vi "disable error reporting.vi"(8 "error in":errorcluster, 10 "module ID":string, 11 "Standard Engine Configuration in":refnum<class "Standard Engine Configuration.lvclass">) -> (0 "error out":errorcluster, 3 "Standard Engine Configuration out":refnum<class "Standard Engine Configuration.lvclass">)   [LabVIEW 2013, in "Standard Engine Configuration.lvclass"]
doc: "Undos the actions taken by the 'enable error reporting.vi'."
uses:
  Standard Engine Configuration.lvclass
  <vilib>/NI/Configuration Framework/serializable configuration/NISE_CEF_serializable configuration.lvclass/NISE_CEF_serializable configuration.ctl
  Standard Engine Configuration.lvclass/Standard Engine Configuration.ctl
  <vilib>/Utility/LVClass/Get LV Class Name.vi
  <vilib>/NI/Module Execution Interface/Engine Configuration/engine configuration.lvclass
  <vilib>/NI/Configuration Framework/serializable configuration/NISE_CEF_serializable configuration.lvclass
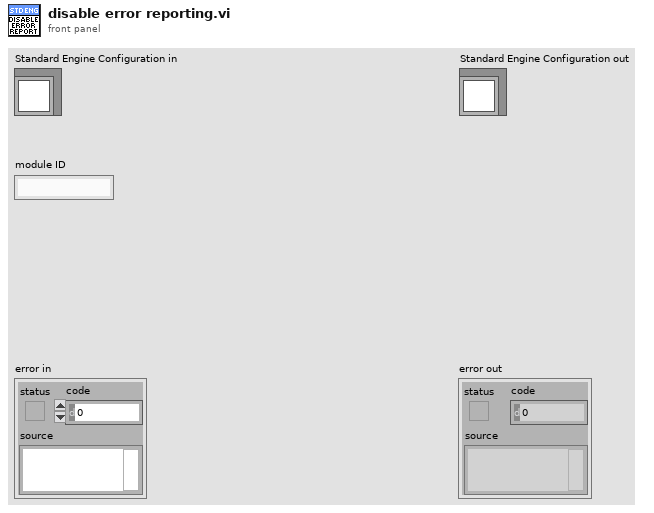
[diagram p1: front panel]
types:
  T1 = typedef "Standard Engine Configuration.lvclass/Module Specific Configuration.ctl" = cluster{"Module ID":string, "Module Decimation":T2, "error tag":string, "error responses":T3, "Initialize on Error?":bool}
  T2 = typedef "Standard Engine Configuration.lvclass/Module Decimation.ctl" = cluster{"Decimation":u16, "Offset":u16, "sort order":i32, "async?":bool}
  T3 = typedef "Standard Engine Configuration.lvclass/error responses.ctl" = cluster{"unknown":T4, "trivial":T4, "critical":T4, "recoverable":T4}
  T4 = typedef "Standard Engine Configuration.lvclass/error options.ctl" = cluster{"clear":bool, "notify":bool, "log":bool, "remove module":bool, "abort engine":bool, "go to safe state":bool, "recover module":bool}
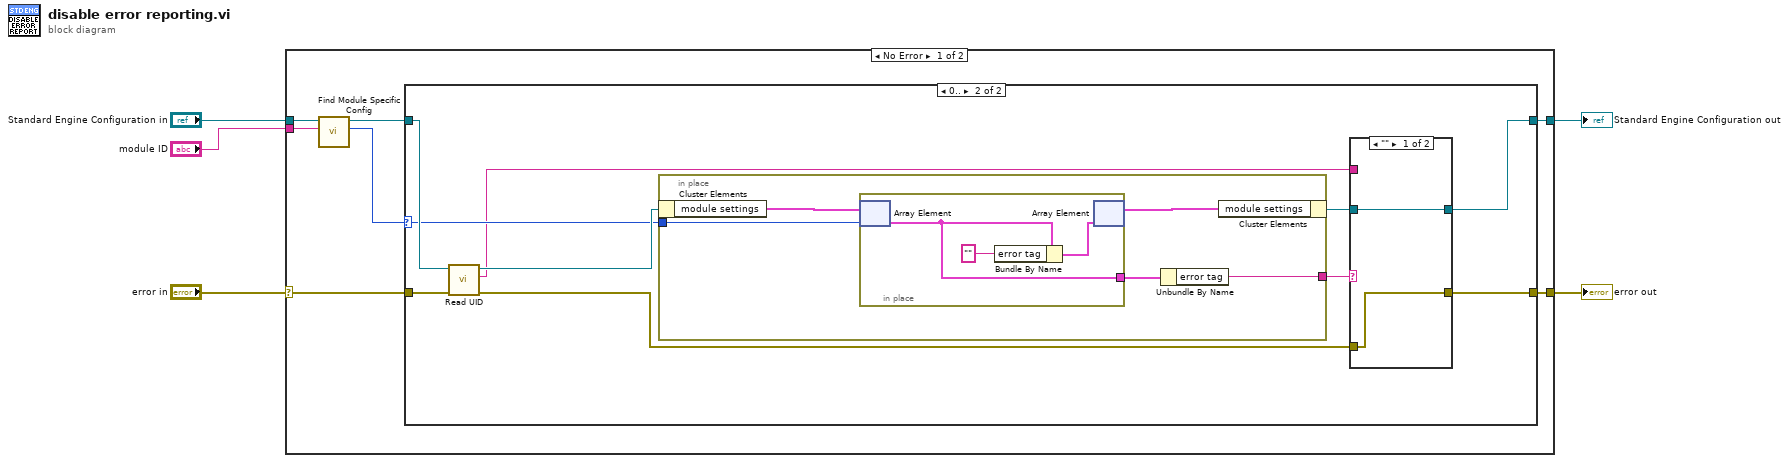
[diagram p0: block diagram]
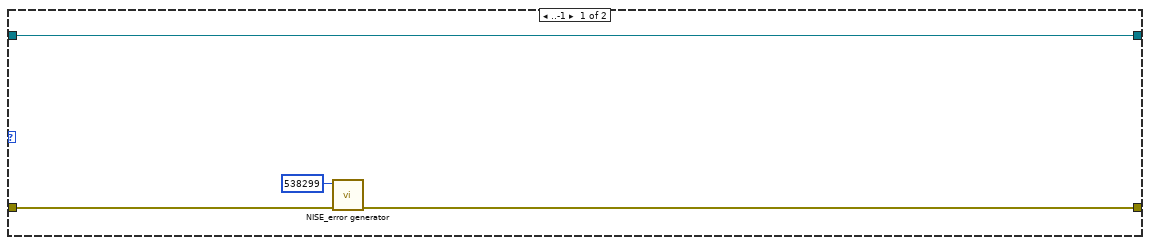
[diagram p2: hidden frame]
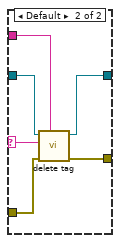
[diagram p3: hidden frame]
diagram:
  n1 = case shown="No Error" "error in" {
    selector: "error in" -> [w8 w44]
    tunnel: "Standard Engine Configuration in" -> [w12 w43]
    tunnel: "module ID" -> [w11 _]
    tunnel: [w6 w43] -> w2
    tunnel: [w7 w44] -> w1
    frame No Error {
      n2 = call "Find Module Specific Config.vi"("Module ID"=w11, "Standard Engine Repo Data in"=w12) -> ("Index"=w9:i32, "Standard Engine Repo Data out"=w10:refnum<class "Standard Engine Configuration.lvclass">)  [unwired: 8 in]
      n3 = case shown="0.." w9 {
        selector: w9 -> [_ w20]
        tunnel: w10 -> [w16 w24]
        tunnel: w8 -> [w15 w26]
        tunnel: [w14 w21] -> w7
        tunnel: [w16 w22] -> w6
        frame ..-1 {
          n4 = call <vilib>:"NISE_error generator.vi"("error in"=w15, "error code (0)"=538299) -> ("error out"=w14:errorcluster)  [unwired: 7 in]
        }
        frame 0.. {
          n5 = call <vilib>:"Read UID.vi"("error in"=w26, "configuration in"=w24) -> ("error out"=w25:errorcluster, "instance id"=w19:string, "configuration out"=w23:refnum<class "Standard Engine Configuration.lvclass">)  [unwired: 7 in]
          n6 = in-place {
            in-place-border: w20 -> [w37]
            in-place-border: [w35] -> w17
            n7 = in-place-cluster #1(w23) -> ("module settings"=w39:T1[])
            n8 = in-place {
              in-place-border: [w41] -> w36
              n9 = in-place-array #2(w39, w37) -> (w41:T1)
              n10 = Bundle By Name(cluster=w41, "error tag"="") -> (w42:T1)
              n11 = in-place-array #2(w42) -> (w38:T1[])  [unwired: 1 out]
            }
            n12 = Unbundle By Name(w36) -> ("error tag"=w35:string)
            n13 = in-place-cluster #1("module settings"=w38) -> (w18:refnum<class "Standard Engine Configuration.lvclass">)
          }
          n14 = case shown="\"\"" w17 {
            selector: w17 -> [_ w29]
            tunnel: w18 -> [w28 w34]
            tunnel: [w28 w33] -> w22
            tunnel: [w27 w32] -> w21
            tunnel: w25 -> [w27 w31]
            tunnel: w19 -> [_ w30]
            frame "" {
            }
            frame Default {
              n15 = call <vilib>:"delete tag.vi"("owner ID"=w30, "error in"=w31, "tag name"=w29, "engine configuration in"=w34) -> ("error out"=w32:errorcluster, "engine configuration out"=w33:refnum<class "Standard Engine Configuration.lvclass">)  [unwired: 6 in]
            }
          }
        }
      }
    }
    frame Error {
    }
  }
  "error out" <- w1
  "Standard Engine Configuration out" <- w2
